vi "FPGA_driver.vi"() -> ()   [LabVIEW 2019]
uses:
  <vilib>/Platform/TimedLoop/XDataNode/timing_clust.ctl
  <vilib>/Platform/TimedLoop/XDataNode/nitl_modes.ctl
  <vilib>/Platform/TimedLoop/XDataNode/wakeup.ctl
  <vilib>/rvi/Emulation/niFpgaGetClockAttributes.vi
  <vilib>/rvi/Emulation/niFpgaSctlEmulationGetInTimedLoop.vi
  <vilib>/rvi/Emulation/niFpgaEmulationReportErrorSimple.vi
  <vilib>/rvi/Emulation/niFpgaProcessEmulError.vi
  <vilib>/rvi/Emulation/niFpgaCriticalErrorInLSC.vi
  <vilib>/rvi/eio/common/nirviEmuTemplateMethod_errors.vi
  <vilib>/rvi/Analysis/common/FxpNativeNode/niFpgaFxpNative.xnode
  <vilib>/eio/EIONode/EIONode.xnode
  <vilib>/platform/TimedLoop/XDataNode/XDataNode.xnode
  <vilib>/Platform/TimedLoop/XDataNode/XDNodeRunTimeDep.lvlib
panel:
  out "ConnectorC/DIO1":bool
  out "ConnectorC/DIO0":bool
  in  "Coil Current Direction":bool
  in  "Num_cycle_on":u32
  in  "enable?":bool
  out "Encoder Position 2":i16
  in  "Encoder Reload Value 2":i16
  out "clk/pulse":i32
  out "Velocity\nValid?":bool
  in  "Position Ref.":i32
  in  "Num Clocks\nper Period":u32=400000
  in  "Velocity \nLimit":i32=10
  in  "Position Loop\nPeriod (ms)":u32=10
  out "Encoder Position":i16
  in  "Encoder Reload Value":i16
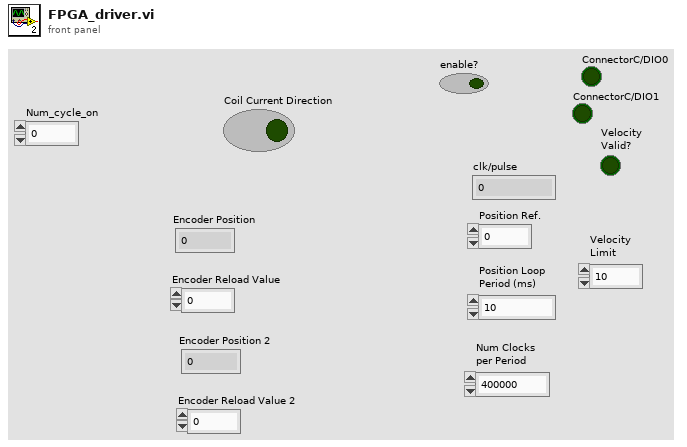
[diagram p1: front panel]
types:
  T1 = typedef "XDNodeRunTimeDep.lvlib/timing_clust.ctl" = cluster{"Expected End [f-1]":u64, "Actual End [f-1]":u64, "Finished Late? [f-1]":bool, "Expected End [i-1]":u64, "Actual End [i-1]":u64, "Finished Late? [i-1]":bool, "Expected Start [i]":u64, "Actual Start [i]":u64, "Expected Start [f]":u64, "Actual Start [f]":u64, "Source Name":string, "Structure Name":string, "Period":i64, "Deadline":i64, "Offset":i64, "Start":i64, "Priority":i32, "Timeout":i32, "Mode":T2, "Wakeup Reason":T3, "Error":errorcluster, "Source Type":string, "Secondary Source Type":string, "Global End Time":u64, "Global Start Time":u64, "Frame Duration":u64, "Iteration Duration":u64, "Assigned CPU":i32, "I/O Scan Engine Mode":u32}
  T2 = typedef "XDNodeRunTimeDep.lvlib/nitl_modes.ctl" = enum32{"No Change", "Process missed periods, maintain original phase", "Discard missed periods, maintain original phase", "Process missed periods, ignore original phase", "Discard missed periods, ignore original phase"}
  T3 = typedef "XDNodeRunTimeDep.lvlib/wakeup.ctl" = enum32{"Normal", "Aborted", "Asynchronous wakeup", "Timing source error", "Timed loop error", "Timeout"}
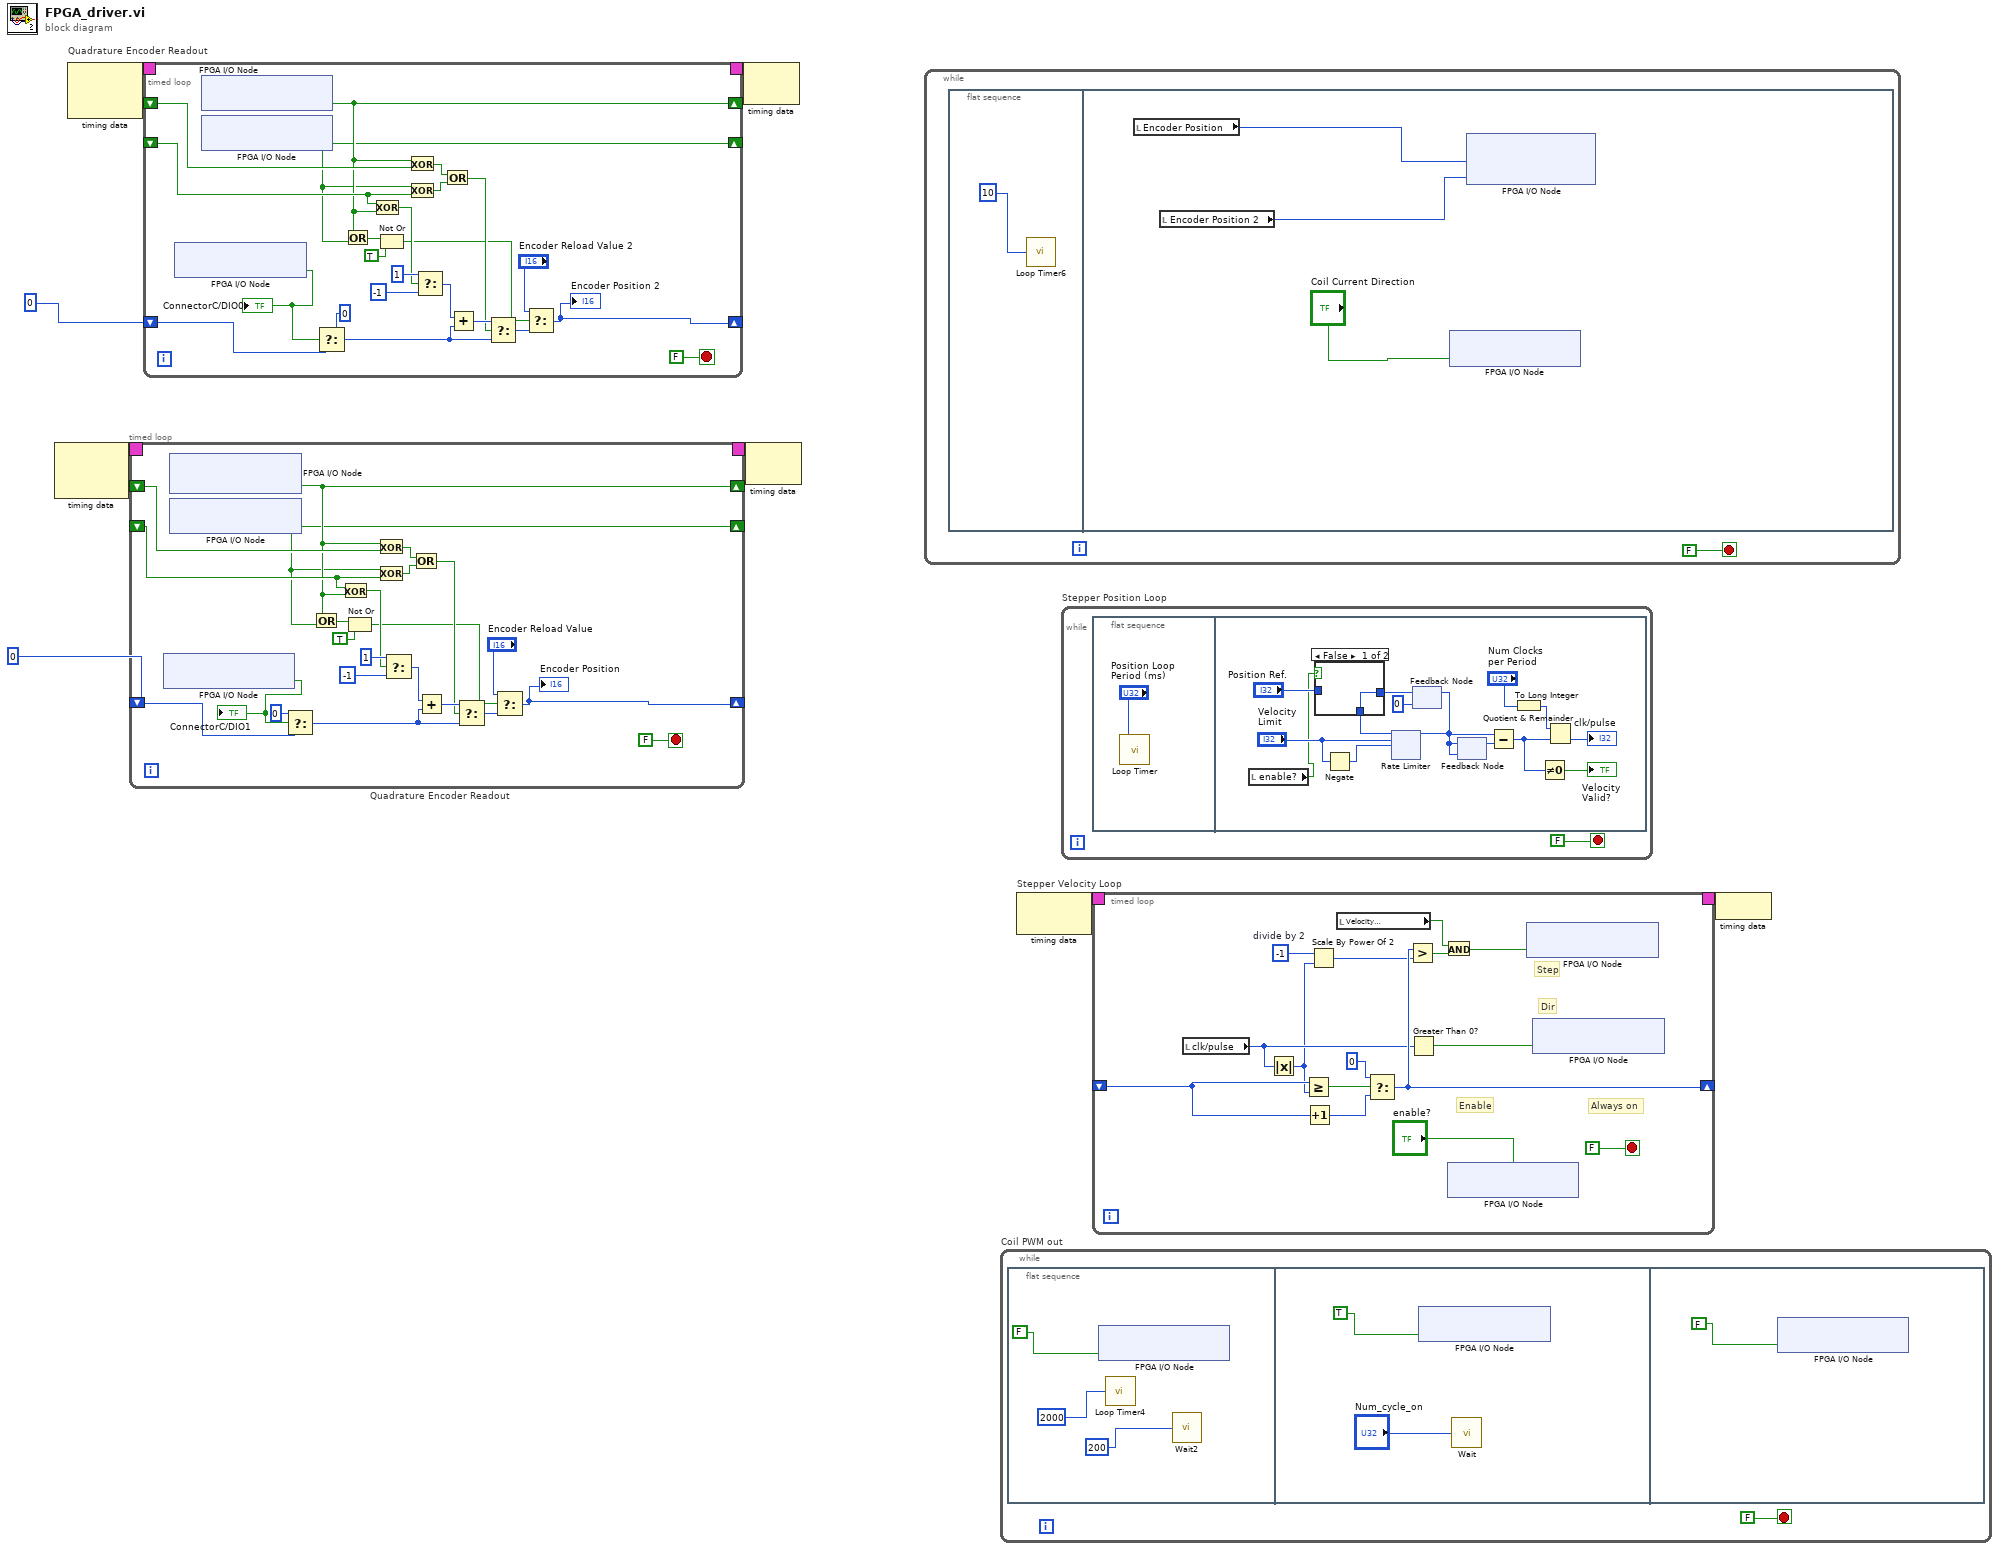
[diagram p0: block diagram]
diagram:
  n1 = node-c288() -> (w8:T1)  [unwired: 2 out]
  n2 = node-c288() -> (w3:T1)  [unwired: 2 out]
  n3 = timed-loop "Quadrature Encoder Readout" {
    timing-out: [_] -> w7
    timing: w8 -> [_]
    shift-left: _ -> [w17]
    shift-right: [w13] -> _
    shift-left: i16 0 -> [w28]
    shift-right: [w10] -> _
    shift-left: _ -> [w18]
    shift-right: [w14] -> _
    stop <- FALSE stop-if-true
    n4 = xnode "FPGA I/O Node"() -> ("ConnectorC/DIO1"=w9:bool)  [unwired: 1 in, 1 out]
    "ConnectorC/DIO1" <- w9
    n5 = xnode "FPGA I/O Node"() -> ("ConnectorA/DIO0"=w14:bool)  [unwired: 2 in, 2 out]
    n6 = xnode "FPGA I/O Node"() -> ("ConnectorA/DIO1"=w13:bool)  [unwired: 1 in, 1 out]
    n7 = Select(t=i16 0, s=w9, f=w28) -> (s? t:f=w29:i16)
    n8 = Or(x=w14, y=w13) -> (x .or. y?=w12:bool)
    n9 = Exclusive Or(1:w14, 2:w17) -> (0:w19:bool)
    n10 = Not Or(1:TRUE ("y"), 2:w12) -> (0:w16:bool)
    n11 = Exclusive Or(1:w18, 2:w14) -> (0:w21:bool)
    n12 = Exclusive Or(1:w17, 2:w13) -> (0:w22:bool)
    n13 = Select(t=i16 1, s=w19, f=i16 -1) -> (s? t:f=w27:i16)
    n14 = Or(x=w21, y=w22) -> (x .or. y?=w20:bool)
    n15 = Add(x=w27, y=w29) -> (x+y=w31:i16)
    n16 = Select(t=w31, s=w20, f=w29) -> (s? t:f=w24:i16)
    n17 = Select(t="Encoder Reload Value", s=w16, f=w24) -> (s? t:f=w10:i16)
    "Encoder Position" <- w10
  }
  n18 = timed-loop "Quadrature Encoder Readout" {
    timing-out: [_] -> w2
    timing: w3 -> [_]
    shift-left: _ -> [w42]
    shift-right: [w38] -> _
    shift-left: i16 0 -> [w53]
    shift-right: [w35] -> _
    shift-left: _ -> [w43]
    shift-right: [w39] -> _
    stop <- FALSE stop-if-true
    n19 = xnode "FPGA I/O Node"() -> ("ConnectorC/DIO0"=w34:bool)  [unwired: 1 in, 1 out]
    "ConnectorC/DIO0" <- w34
    n20 = xnode "FPGA I/O Node"() -> ("ConnectorA/DIO2"=w39:bool)  [unwired: 1 in, 1 out]
    n21 = xnode "FPGA I/O Node"() -> ("ConnectorA/DIO3"=w38:bool)  [unwired: 1 in, 1 out]
    n22 = Select(t=i16 0, s=w34, f=w53) -> (s? t:f=w54:i16)
    n23 = Or(x=w39, y=w38) -> (x .or. y?=w37:bool)
    n24 = Exclusive Or(1:w39, 2:w42) -> (0:w44:bool)
    n25 = Not Or(1:TRUE ("y"), 2:w37) -> (0:w41:bool)
    n26 = Exclusive Or(1:w43, 2:w39) -> (0:w46:bool)
    n27 = Exclusive Or(1:w42, 2:w38) -> (0:w47:bool)
    n28 = Select(t=i16 1, s=w44, f=i16 -1) -> (s? t:f=w52:i16)
    n29 = Or(x=w46, y=w47) -> (x .or. y?=w45:bool)
    n30 = Add(x=w52, y=w54) -> (x+y=w56:i16)
    n31 = Select(t=w56, s=w45, f=w54) -> (s? t:f=w49:i16)
    n32 = Select(t="Encoder Reload Value 2", s=w41, f=w49) -> (s? t:f=w35:i16)
    "Encoder Position 2" <- w35
  }
  n33 = node-c288(w2) -> ()  [unwired: 1 out]
  n34 = node-c288(w7) -> ()  [unwired: 1 out]
  n35 = while {
    stop <- FALSE stop-if-true
    n36 = flat-sequence {
      frame #0 {
        n37 = call "Loop Timer6"("Count(mSec)"=u32 10) -> ()  [unwired: 1 out]
      }
      frame #1 {
        n38 = local read "Encoder Position"() -> (w62:i16)
        n39 = local read "Encoder Position 2"() -> (w63:i16)
        n40 = xnode "FPGA I/O Node"("ConnectorC/DIO0"="Coil Current Direction") -> ()  [unwired: 1 in, 1 out]
        n41 = xnode "FPGA I/O Node"("ConnectorC/AO0"=w62, "ConnectorC/AO1"=w63) -> ()  [unwired: 2 in, 2 out]
      }
    }
  }
  n42 = while "Coil PWM out" {
    stop <- FALSE stop-if-true
    n43 = flat-sequence {
      frame #0 {
        n44 = xnode "FPGA I/O Node"("ConnectorC/DIO1"=FALSE) -> ()  [unwired: 1 in, 1 out]
        n45 = call "Loop Timer4"("Count(Ticks)"=u32 2000 ("Count(uSec)")) -> ()  [unwired: 1 out]
        n46 = call "Wait2"("Count(Ticks)"=u32 200) -> ()  [unwired: 1 out]
      }
      frame #1 {
        n47 = xnode "FPGA I/O Node"("ConnectorC/DIO1"=TRUE) -> ()  [unwired: 1 in, 1 out]
        n48 = call "Wait"("Count(Ticks)"="Num_cycle_on") -> ()  [unwired: 1 out]
      }
      frame #2 {
        n49 = xnode "FPGA I/O Node"("ConnectorC/DIO1"=FALSE) -> ()  [unwired: 1 in, 1 out]
      }
    }
  }
  n50 = node-c288() -> (w5:T1)  [unwired: 1 in]
  n51 = while "Stepper Position Loop" {
    stop <- FALSE stop-if-true
    n52 = flat-sequence {
      frame #0 {
        n53 = call "Loop Timer"("Count(mSec)"="Position Loop\nPeriod (ms)") -> ()  [unwired: 1 out]
      }
      frame #1 {
        n54 = local read "enable?"() -> (w73:bool)
        n55 = Negate(x="Velocity \nLimit") -> (-x=w80:i32)
        n56 = feedback #1(0 ("output")) -> (w75:i32)
        n57 = case shown="False" w73 {
          tunnel: [w87 w88] -> w78
          tunnel: "Position Ref." -> [_ w88]
          tunnel: w75 -> [w87 _]
          frame False {
          }
          frame True {
          }
        }
        n58 = xnode ("Rate Limiter")("pos slew rate * dt"="Velocity \nLimit", "input"=w78, "neg slew rate * dt"=w80) -> ("output"=w76:i32)  [unwired: 1 in]
        n59 = feedback-in #1(w76) -> ()
        n60 = feedback #2(w76) -> (w85:i32)
        n61 = feedback-in #2(w76) -> ()
        n62 = Subtract(x=w76, y=w85) -> (x-y=w82:i32)
        n63 = To Long Integer(number="Num Clocks\nper Period") -> (32bit integer=w83:i32)
        n64 = Not Equal To 0?(x=w82) -> (x != 0?=→"Velocity\nValid?":bool)
        n65 = Quotient & Remainder(x=w83, y=w82) -> (floor(x/y)=→"clk/pulse":i32)  [unwired: 1 out]
      }
    }
  }
  n66 = timed-loop "Stepper Velocity Loop" {
    timing: w5 -> [_]
    timing-out: [_] -> w4
    shift-right: [w123] -> _
    shift-left: _ -> [w120]
    stop <- FALSE stop-if-true
    w116 = -1  # divide by 2
    # "Always on"
    # "Enable"
    # "Dir"
    # "Step"
    n67 = local read "clk/pulse"() -> (w119:i32)
    n68 = Absolute Value(x=w119) -> (abs(x)=w117:i32)
    n69 = Greater Or Equal?(x=w120, y=w117) -> (x >= y?=w124:bool)
    n70 = Increment(x=w120) -> (x+1=w126:i32)
    n71 = Scale By Power Of 2(n=w116, x=w117) -> (x*2^n=w118:i32)
    n72 = local read "Velocity\nValid?"() -> (w121:bool)
    n73 = Select(t=0, s=w124, f=w126) -> (s? t:f=w123:i32)
    n74 = Greater?(x=w123, y=w118) -> (0:w122:bool)
    n75 = Greater Than 0?(x=w119) -> (x > 0?=w115:bool)
    n76 = And(x=w121, y=w122) -> (x .and. y?=w114:bool)
    n77 = xnode "FPGA I/O Node"("ConnectorC/DIO4"="enable?") -> ()  [unwired: 1 in, 1 out]
    n78 = xnode "FPGA I/O Node"("ConnectorC/DIO2"=w114) -> ()  [unwired: 1 in, 1 out]
    n79 = xnode "FPGA I/O Node"("ConnectorC/DIO3"=w115) -> ()  [unwired: 1 in, 1 out]
  }
  n80 = node-c288(w4) -> ()
